vi "PFI-28000-Utils_Parse Help.vi"(0 "String":string, 5 "Command":string, 11 "error in (no error)":errorcluster) -> (4 "Options":string[](array[string]), 15 "error out":errorcluster)   [LabVIEW 2017, in "PFI-28000-Utils.lvlib"]
uses:
  PFI-28000-Utils.lvlib
  <vilib>/regexp/Match Regular Expression.xnode
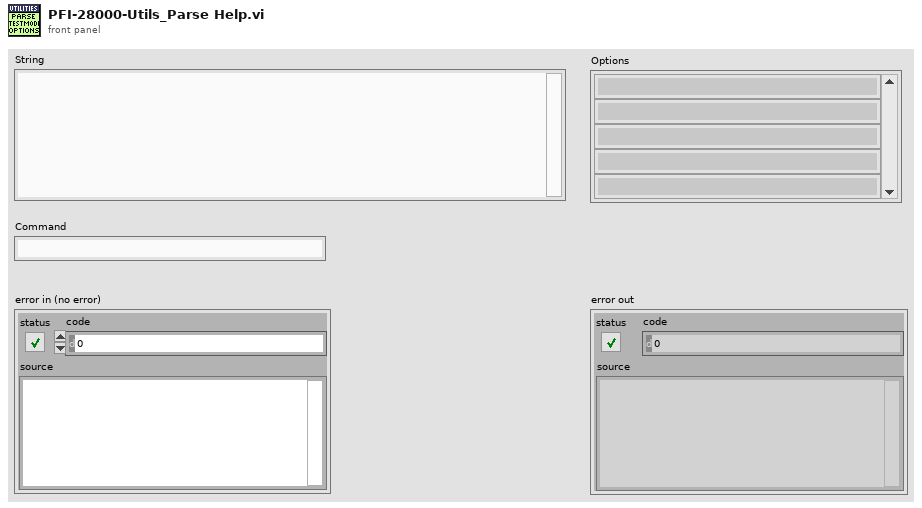
[diagram p1: front panel]
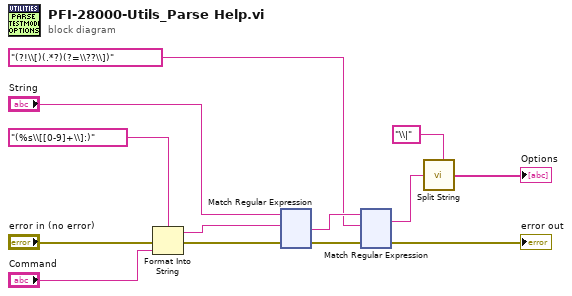
[diagram p0: block diagram]
diagram:
  n1 = Format Into String(format string="(%s\\[[0-9]+\\]:)" ("empty string"), error in="error in (no error)", "Command") -> (resulting string=w3:string, error out=w1:errorcluster)  [unwired: 1 in]
  n2 = xnode "Match Regular Expression"("input string"="String", "regular expression"=w3, "error in"=w1) -> ("after match"=w12:string, "error out"=w7:errorcluster)  [unwired: 3 in, 3 out]
  n3 = xnode "Match Regular Expression"("input string"=w12, "regular expression"="(?!\\[)(.*?)(?=\\??\\])" ("empty string"), "error in"=w7) -> ("whole match"=w10:string, "error out"=→"error out":errorcluster)  [unwired: 3 in, 3 out]
  n4 = call <vilib>:"Split String.vi"("Split Pattern"="\\|" ("empty string"), "Input String"=w10) -> ("Split String"=→"Options":string[])  [unwired: 5 in]
